vi "Data handler-Live imaging protocol.vi"(0 "Image array":T7, 1 "Logging queue":refnum<queue>, 5 "Logging queue element in":T3={"Imaging Protocol"=enum."Live Imaging", "Number of Trials"=0, "Frame Size"=512, "# Averaged frames"=0, "Dwell time (us)"=0.0, "Index of Z-plane"=0, "Timelapse?"=FALSE, "Logging process is active"=FALSE, "Speed logging enabled"=FALSE, "tdms file ref"=refnum, "path"=path "", "Trial Number"=0, "Expected # points acquired"=FALSE, "Manually stopped"=FALSE, "Last trial"=FALSE, "Ch0 data"=[], "Ch1 data"=[], "Image Time"=[], "Continuous Time"=[], "Points acquired"={"Ch0 last trial"=0, "Ch1 last trial"=0, "All trials"=0}, "HW Timings File"=refnum} {"Frame Size" items=["100X100"=100, "128X128"=128, "200X200"=200, "256X256"=256, "512X512"=512, "1024x1024"=1024, "2048x2048"=2048]; "Dwell time (us)" format="%#.6g"}, 9 "Live graph data queue in":T2, 11 "error in (no error)":errorcluster, 12 "Single Frame Data":T1, 13 "Frame completed/generate image":bool) -> (15 "error out":errorcluster)   [LabVIEW 2017]
uses:
  User Interface/Queue/Live graphs queue/Typedefs/Live imaging queue element.ctl
  <vilib>/vision/Image Controls.llb/IMAQ Image.ctl
  Typedefs/Logging queue element.ctl
  Typedefs/Imaging Protocols enum.ctl
  Typedefs/Frame Size.ctl
  Typedefs/Acquired points count.ctl
  User Interface/Typedefs/Live graph data queue ref.ctl
  Typedefs/Frame data dual cluster.ctl
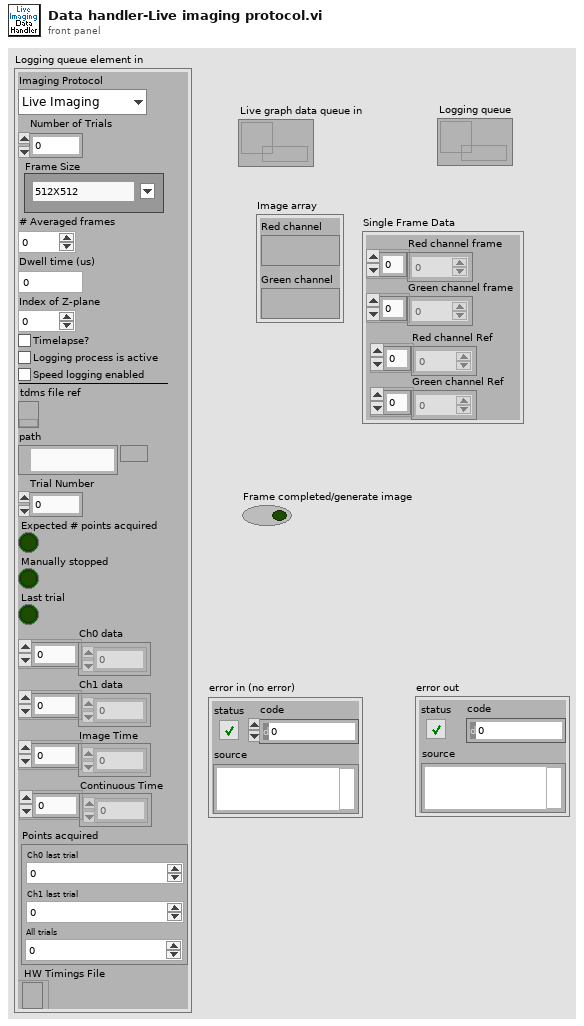
[diagram p1: front panel]
types:
  T1 = typedef "Frame data dual cluster.ctl" = cluster{"Red channel frame":dbl[], "Green channel frame":dbl[], "Red channel Ref":dbl[], "Green channel Ref":dbl[]}
  T2 = typedef "Live graph data queue ref.ctl" = refnum<queue>
  T3 = typedef "Logging queue element.ctl" = cluster{"Imaging Protocol":T4, "Number of Trials":u16, "Frame Size":T5, "# Averaged frames":u16, "Dwell time (us)":dbl, "Index of Z-plane":i32, "Timelapse?":bool, "Logging process is active":bool, "Speed logging enabled":bool, "tdms file ref":refnum<k34>, "path":path, "Trial Number":i32, "Expected # points acquired":bool, "Manually stopped":bool, "Last trial":bool, "Ch0 data":u32[], "Ch1 data":u32[], "Image Time":u64[], "Continuous Time":u64[], "Points acquired":T6, "HW Timings File":refnum<file>}
  T4 = typedef "Imaging Protocols enum.ctl" = enum16{"AOL Z-Stack", "Motor Z Stack", "Functional Acquisition", "Single Plane Acquisition", "Volume Acquisition", "Live Imaging", "Live Plane Imaging", "Live Volume Imaging"}
  T5 = typedef "Frame Size.ctl" = u16
  T6 = typedef "Acquired points count.ctl" = cluster{"Ch0 last trial":u64, "Ch1 last trial":u64, "All trials":u64}
  T7 = typedef "Live imaging queue element.ctl" = cluster{"Red channel":T8, "Green channel":T8}
  T8 = typedef "IMAQ Image.ctl" = refnum<image>
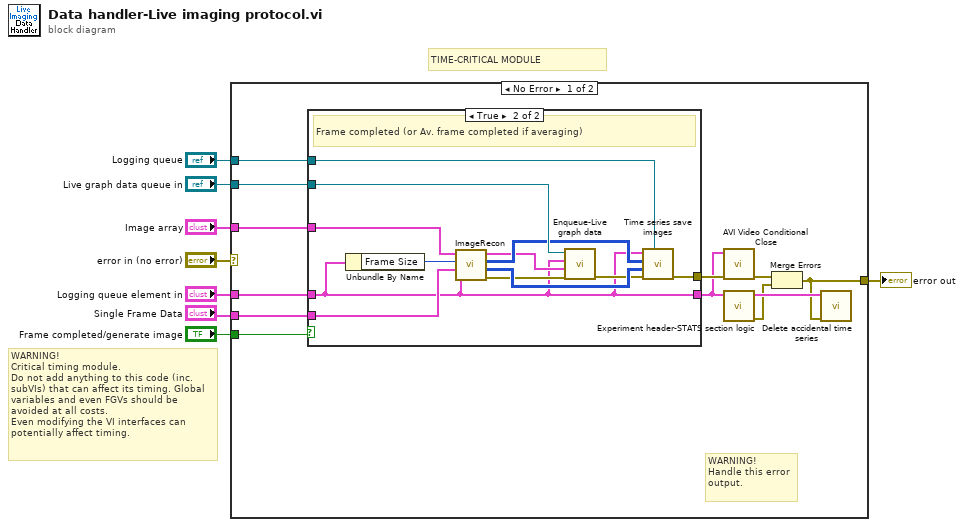
[diagram p0: block diagram]
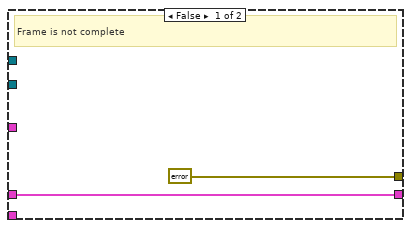
[diagram p2: hidden frame]
diagram:
  # "TIME-CRITICAL MODULE"
  # "WARNING!\nCritical timing module.\nDo not add anything to this code (inc. subVIs) that can affect its timing. Global variables and even FGVs should be avoided at all costs.\nEven modifying the VI interfaces can potentially affect timing."
  n1 = case shown="No Error" "error in (no error)" {
    selector: "error in (no error)" -> [_ w34]
    tunnel: [w9 w34] -> w8
    tunnel: "Image array" -> [w16 _]
    tunnel: "Logging queue element in" -> [w13 _]
    tunnel: "Live graph data queue in" -> [w17 _]
    tunnel: "Frame completed/generate image" -> [w19 _]
    tunnel: "Single Frame Data" -> [w15 _]
    tunnel: "Logging queue" -> [w18 _]
    frame No Error {
      # "WARNING!\nHandle this error\noutput."
      n2 = case shown="True" w19 {
        tunnel: w16 -> [_ w33]
        tunnel: [errorcluster {"status"=FALSE, "code"=0, "source"=""} ("error out") w25] -> w14
        tunnel: w13 -> [w20 w22]
        tunnel: w15 -> [_ w32]
        tunnel: w17 -> [_ w31]
        tunnel: w18 -> [_ w23]
        tunnel: [w20 w22] -> w12
        frame False {
          # "Frame is not complete"
        }
        frame True {
          # "Frame completed (or Av. frame completed if averaging)"
          n3 = Unbundle By Name(w22) -> ("Frame Size"=w30:T5)
          n4 = call "ImageRecon.vi"("Logging queue element in"=w22, "Data"=w32, "Frame Size"=w30, "Image Array (in)"=w33) -> ("Error Out"=w27:errorcluster, "Ch1-Green"=w28:i16[][], "Ch0-Red"=w29:i16[][], "Image Array(out)"=w24:T7)  [unwired: 4 in]
          n5 = call "Enqueue-Live graph data.vi"("error in (no error)"=w27, "Element to queue"=w24, "Logging queue element"=w22, "Live graph data queue in"=w31) -> ("error out"=w26:errorcluster)  [unwired: 6 in, 1 out]
          n6 = call "Time series save images.vi"("Logging queue"=w23, "error in (no error)"=w26, "Ch1-Green"=w28, "Ch0-Red"=w29, "Logging queue element"=w22) -> ("error"=w25:errorcluster)  [unwired: 6 in]
        }
      }
      n7 = call "AVI Video Conditional Close.vi"("error in (no error)"=w14, "Logging queue element in"=w12) -> ("error out"=w11:errorcluster)  [unwired: 9 in]
      n8 = call "Experiment header-STATS section logic.vi"("Logging queue element"=w12) -> ("error out"=w10:errorcluster)  [unwired: 10 in]
      n9 = Merge Errors(w11, w10) -> (w9:errorcluster)
      n10 = call "Delete accidental time series.vi"("error in (no error)"=w9, "Logging queue element in"=w12) -> ()  [unwired: 10 in]
    }
    frame Error {
    }
  }
  "error out" <- w8
